vi "RT GV.vi"() -> ()   [LabVIEW 2021]
panel:
  in  "Enable P&P?":bool
  in  "Offsets":dbl[](array[numeric])=[0.0, 0.0, 0.0, 0.0]
  out "End Cycle":bool
  in  "Machine Error":string
  in  "Machine Status":string
  out "BF Delays":u32[](array[numeric])=[1000, 1000]
  out "Agitator Delays":u32[](array[numeric])=[400, 5000]
  out "Stop Initiated":bool
  in  "Enable Auto":bool
  in  "Enable BF?":bool
  in  "Enable Agitate?":bool
  in  "Enable Reject?":bool
  in  "Enable Measurement?":bool
  in  "Enable Index?":bool
  in  "Enable PF?":bool
  in  "Enable Cutting?":bool
  in  "Enable Insertion?":bool
  in  "Enable TF?":bool
  in  "Continuous Index?":bool
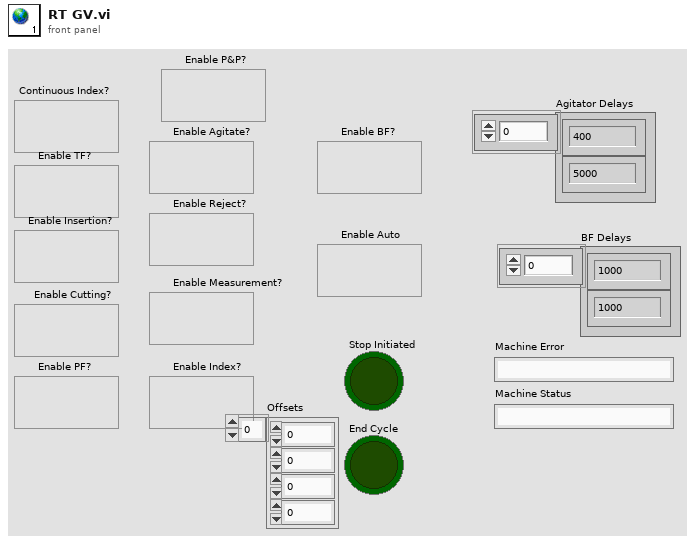
[diagram p1: front panel]
diagram:
